vi "Test TS Environment Manager - Get Installations.vi"() -> (0 "error out":errorcluster)   [LabVIEW 2025]
doc: "Test fetching of installations in the current system (using mock)."
uses:
  src/TSDiscovery Mock/TSDiscovery Mock.lvclass
  src/Type Definitions/TSInstall--cluster.ctl
  src/Type Definitions/Architecture--enum.ctl
  <vilib>/addons/_JKI Toolkits/Caraya/classes/Test/Test.lvclass
  src/Libraries/TS Environment Manager/TS Environment Manager.lvlib
  <vilib>/addons/_JKI Toolkits/Caraya/classes/Assert/Assert.lvclass
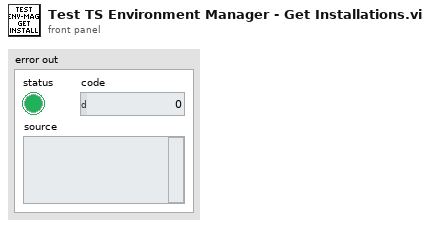
[diagram p1: front panel]
types:
  T1 = typedef "TSInstall--cluster.ctl" = cluster{"Version":string, "Architecture":T2, "Version Key":string, "ID":string}
  T2 = typedef "Architecture--enum.ctl" = enum16{"32bit", "64bit"}
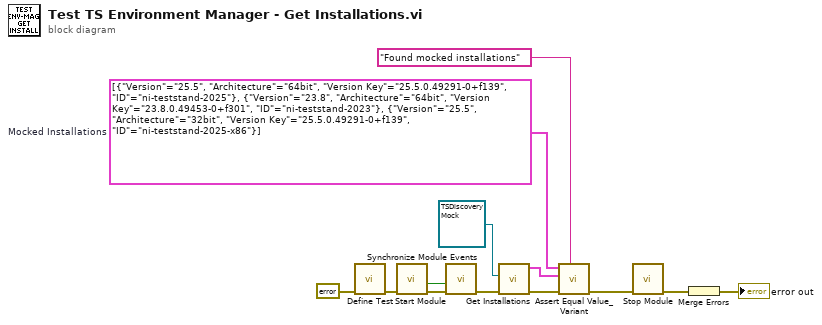
[diagram p0: block diagram]
diagram:
  w7 = T1[] [{"Version"="25.5", "Architecture"=enum."64bit", "Version Key"="25.5.0.49291-0+f139", "ID"="ni-teststand-2025"}, {"Version"="23.8", "Architecture"=enum."64bit", "Version Key"="23.8.0.49453-0+f301", "ID"="ni-teststand-2023"}, {"Version"="25.5", "Architecture"=enum."32bit", "Version Key"="25.5.0.49291-0+f139", "ID"="ni-teststand-2025-x86"}]  # Mocked Installations
  n1 = call <vilib>:"Define Test.vi"("error in (no error)"=errorcluster {"status"=FALSE, "code"=0, "source"=""}) -> ("error out"=w5:errorcluster)  [unwired: 9 in, 1 out]
  n2 = call "Start Module.vi"("error in"=w5) -> ("error out"=w12:errorcluster, "Wait for Event Sync?"=w11:bool)  [unwired: 6 in, 3 out]
  n3 = call "Synchronize Module Events.vi"("error in"=w12, "Wait for Event Sync?"=w11) -> ("error out"=w10:errorcluster)  [unwired: 9 in]
  n4 = call "Get Installations.vi"("error in"=w10, "ITSDiscovery.lvclass"=refnum<class "TSDiscovery Mock.lvclass"> refnum ("TSDiscovery Mock.lvclass")) -> ("error out"=w4:errorcluster, "Installations"=w6:T1[])  [unwired: 7 in, 1 out]
  n5 = call <vilib>:"Assert Equal Value_Variant.vi"("Label"="Found mocked installations" ("Label (VI Title)"), "error in (no error)"=w4, "Actual"=w6, "Expected"=w7) -> ("error out"=w2:errorcluster)  [unwired: 6 in, 1 out]
  n6 = call "Stop Module.vi"("error in"=w2) -> ("error out"=w1:errorcluster)  [unwired: 10 in]
  n7 = Merge Errors(w1) -> (→"error out":errorcluster)
